vi "Comm - Send Email.vi"(5 "Outgoing Mail Server (SMTP)":string, 6 "Sender's Email Address":string, 7 "Port":u16=25, 8 "error in":errorcluster, 9 "Message":string, 10 "Subject":string, 11 "Recipients":string) -> (0 "error out":errorcluster)   [LabVIEW 2013]
doc: "Creates and sends an email according to the settings you specify in the configuration dialog box.\n--------------------\n\nThis Express VI is configured as follows:\n\nThis VI can be used to programmatically send emails"
uses:
  <vilib>/smtpClient/LabVIEWSMTPClient.lvlib
panel:
  in  "Require Log-in":bool
  in  "Use Secure Connection (TLS\\SSL":bool
  in  "Password":string
  in  "Username":string
  # "Refer to the LabVIEW Help,\navailable by selecting\nHelp>Search the\nLabVIEW Help, for\ninformation about\ndesigning \"source VIs\".\n(Include quotes)"
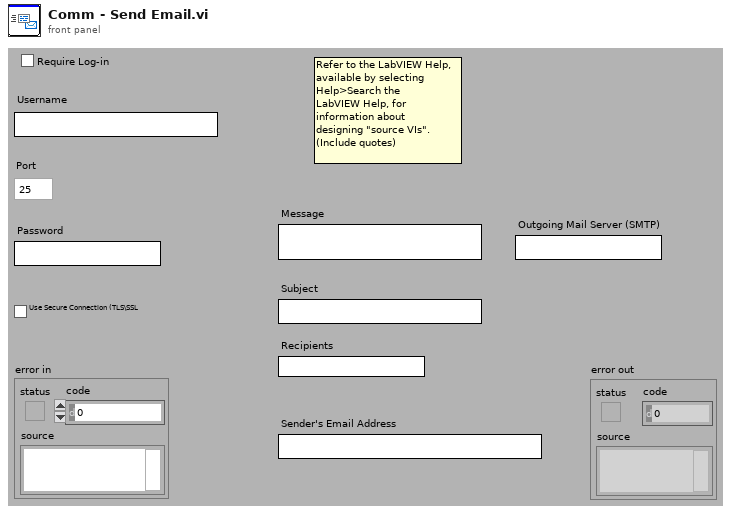
[diagram p1: front panel]
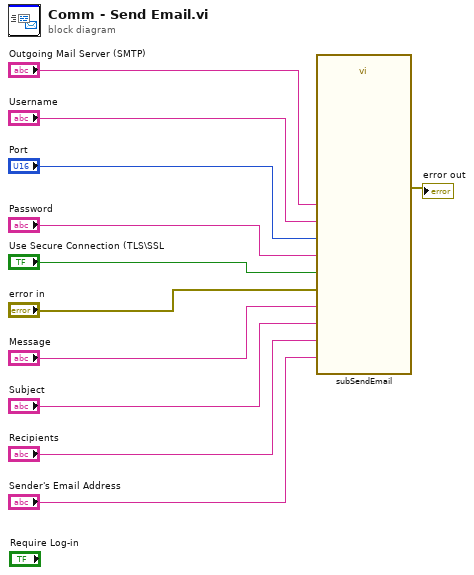
[diagram p0: block diagram]
diagram:
  n1 = call <vilib>:"subSendEmail.vi"("Sender's Email Address"="Sender's Email Address", "Recipients"="Recipients", "Subject"="Subject", "Message"="Message", "error in (no error)"="error in", "Use Secure Connection (TLS\\SSL"="Use Secure Connection (TLS\\SSL", "Password"="Password", "Port"="Port", "Username"="Username", "Outgoing Mail Server (SMTP)"="Outgoing Mail Server (SMTP)") -> ("error out"=→"error out":errorcluster)  [unwired: 9 in]
